vi "VI CG-Check Konfig.vi"() -> ()   [LabVIEW 2020, in "Erweiterte Konfig.lvlib" / "CG-Check Konfig.lvlib"]
uses:
  CG-Check Konfig.lvlib
  Sollwerte_CG-Check.ctl
  Komponenten.ctl
  maxAbweichung_CG-Check.ctl
  Visualisierungs Elemente/Auswahlfeld.ctl
  System Einstellungen V2/Gasflasche Auswahl.ctl
  System Einstellungen V2/Konfig Gasflasche.ctl
  Analysator Definition/FGV Analysator Definition Aktionen.ctl
  System Einstellungen V2/Aktioen FGV System Konstanten.ctl
  System Einstellungen V2/Aktion FGV Gasbottledefinition.ctl
  FT-IR/FGV FT-IR Gasliste Aktionen.ctl
  CalEingaenge.ctl
  Aktion_CG-Check.ctl
  CG-Test.vi
  FT-IR/FT-IR.lvlib
  Allgemein/allgemeine Sub-VIs.lvlib
  Analysator Definition/Analysator Definition.lvlib
  Sprachverwaltung/Sprachverwaltung.lvlib
  System Einstellungen V2/System Einstellungen V2.lvlib
panel:
  in  "Start":bool
  in  "Auswertung":bool caption="Ergebnis"
  in  "Textname:":string
  in  "Pfad:":path=path "D:/IAG_Data/Log" caption="Pfad CalGas Test:"
  in  "Cluster":T1={"Aufschaltdauer"=0.0, "Prüfdauer"=0.0, "Mittelwertanzahl"=10} {"Prüfdauer" format="%#_5g"; "Aufschaltdauer" format="%#_5g"}
  in  "CalGas Konfig":T2(tab)
  in  "Konfig Gasflasche 1":T3 caption="Konfigurierte Gasflasche verwenden"
  in  "Gasflasche 1":T4 caption="Gasflasche" items=["----"=10000]
  in  "Analysator 1":T5 caption="Analysator"
  in  "über PNS":bool
  in  "Komponenten 1":T6 caption="Komponente" {"Komponente 5" items=["---"]; "Komponente 4" items=["---"]; "Komponente 3" items=["---"]; "Komponente 2" items=["---"]; "Komponente 1" items=["---"]}
  in  "Sollwerte 1":T7 caption="Sollwert" {"Sollwert 5" format="%#_10f"; "Sollwert 4" format="%#_10f"; "Sollwert 3" format="%#_10f"; "Sollwert 2" format="%#_10f"; "Sollwert 1" format="%#_10f"}
  in  "max. Abweichung 1":T8 caption="max. Abweichung" {"Abweichung 5" format="%#_5g"; "Abweichung 4" format="%#_5g"; "Abweichung 3" format="%#_5g"; "Abweichung 2" format="%#_5g"; "Abweichung 1" format="%#_5g"}
  in  "Span 1 durchführen":bool
  in  "Konfig Gasflasche 2":T3 caption="Konfigurierte Gasflasche verwenden"
  in  "Gasflasche 2":T4 caption="Gasflasche" items=["----"=10000]
  in  "über PNS":bool
  in  "Sollwerte 2":T7 caption="Sollwert" {"Sollwert 5" format="%#_10f"; "Sollwert 4" format="%#_10f"; "Sollwert 3" format="%#_10f"; "Sollwert 2" format="%#_10f"; "Sollwert 1" format="%#_10f"}
  in  "Komponenten 2":T6 caption="Komponente" {"Komponente 5" items=["---"]; "Komponente 4" items=["---"]; "Komponente 3" items=["---"]; "Komponente 2" items=["---"]; "Komponente 1" items=["---"]}
  in  "max. Abweichung 2":T8 caption="max. Abweichung" {"Abweichung 5" format="%#_5g"; "Abweichung 4" format="%#_5g"; "Abweichung 3" format="%#_5g"; "Abweichung 2" format="%#_5g"; "Abweichung 1" format="%#_5g"}
  in  "Span 2 durchführen":bool
  in  "Analysator 2":T5 caption="Analysator"
  in  "Konfig Gasflasche 3":T3 caption="Konfigurierte Gasflasche verwenden"
  in  "Gasflasche 3":T4 caption="Gasflasche" items=["----"=10000]
  in  "Sollwerte 3":T7 caption="Sollwert" {"Sollwert 5" format="%#_10f"; "Sollwert 4" format="%#_10f"; "Sollwert 3" format="%#_10f"; "Sollwert 2" format="%#_10f"; "Sollwert 1" format="%#_10f"}
  in  "Komponenten 3":T6 caption="Komponente" {"Komponente 5" items=["---"]; "Komponente 4" items=["---"]; "Komponente 3" items=["---"]; "Komponente 2" items=["---"]; "Komponente 1" items=["---"]}
  in  "max. Abweichung 3":T8 caption="max. Abweichung" {"Abweichung 5" format="%#_5g"; "Abweichung 4" format="%#_5g"; "Abweichung 3" format="%#_5g"; "Abweichung 2" format="%#_5g"; "Abweichung 1" format="%#_5g"}
  in  "über PNS":bool
  in  "Span 3 durchführen":bool
  in  "Analysator 3":T5 caption="Analysator"
  in  "Sollwerte 4":T7 caption="Sollwert" {"Sollwert 5" format="%#_10f"; "Sollwert 4" format="%#_10f"; "Sollwert 3" format="%#_10f"; "Sollwert 2" format="%#_10f"; "Sollwert 1" format="%#_10f"}
  in  "Komponenten 4":T6 caption="Komponente" {"Komponente 5" items=["---"]; "Komponente 4" items=["---"]; "Komponente 3" items=["---"]; "Komponente 2" items=["---"]; "Komponente 1" items=["---"]}
  in  "max. Abweichung 4":T8 caption="max. Abweichung" {"Abweichung 5" format="%#_5g"; "Abweichung 4" format="%#_5g"; "Abweichung 3" format="%#_5g"; "Abweichung 2" format="%#_5g"; "Abweichung 1" format="%#_5g"}
  in  "Cal Gas O2 durchführen":bool
  in  "Abbrechen":bool
  in  "speichern":bool
  in  "über PNS":bool caption="Span 1"
  # "Konfiguration CG-Test"
  # "sec"
  # "sec"
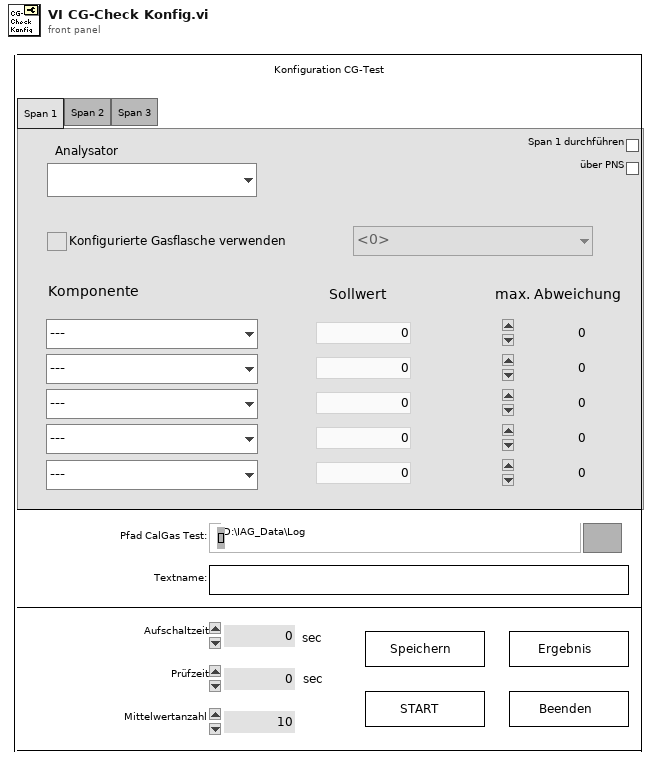
[diagram p1: front panel]
types:
  T1 = cluster{"Aufschaltdauer":sgl, "Prüfdauer":sgl, "Mittelwertanzahl":u8}
  T2 = enum32{"Span 1", "Span 2", "Span 3", "Cal Gas O2"}
  T3 = typedef "System Einstellungen V2.lvlib/Konfig Gasflasche.ctl" = bool
  T4 = typedef "System Einstellungen V2.lvlib/Gasflasche Auswahl.ctl" = u16
  T5 = typedef "Auswahlfeld.ctl" = u16
  T6 = typedef "Erweiterte Konfig.lvlib/CG-Check Konfig.lvlib/Komponenten.ctl" = cluster{"Komponente 1":u16, "Komponente 2":u16, "Komponente 3":u16, "Komponente 4":u16, "Komponente 5":u16}
  T7 = typedef "Erweiterte Konfig.lvlib/CG-Check Konfig.lvlib/Sollwerte_CG-Check.ctl" = cluster{"Sollwert 1":sgl, "Sollwert 2":sgl, "Sollwert 3":sgl, "Sollwert 4":sgl, "Sollwert 5":sgl}
  T8 = typedef "Erweiterte Konfig.lvlib/CG-Check Konfig.lvlib/maxAbweichung_CG-Check.ctl" = cluster{"Abweichung 1":sgl, "Abweichung 2":sgl, "Abweichung 3":sgl, "Abweichung 4":sgl, "Abweichung 5":sgl}
  T9 = typedef "System Einstellungen V2.lvlib/Aktion FGV Gasbottledefinition.ctl" = enum16{"lesen", "schreiben", "löschen", "laden", "speichern", "exportieren", "importieren"}
  T10 = typedef "System Einstellungen V2.lvlib/Aktioen FGV System Konstanten.ctl" = enum16{"lesen", "laden", "speichern", "Sprache"}
  T11 = typedef "Analysator Definition.lvlib/FGV Analysator Definition Aktionen.ctl" = enum16{"lesen", "MB setzen", "MB KAL setzen", "laden"}
  T12 = typedef "Erweiterte Konfig.lvlib/CG-Check Konfig.lvlib/Aktion_CG-Check.ctl" = enum16{"lesen", "schreiben", "laden", "Komponente", "Aktive?", "speichern"}
  T13 = typedef "Erweiterte Konfig.lvlib/CG-Check Konfig.lvlib/CalEingaenge.ctl" = string[]
  T14 = typedef "FT-IR.lvlib/FGV FT-IR Gasliste Aktionen.ctl" = enum16{"lesen", "Gasliste FT-IR", "Gasliste ausgelesen", "laden", "speichern", "löschen"}
  T15 = enum8{"Enabled", "Disabled", "Disabled and Grayed Out"}
  T16 = typedef "System Einstellungen V2.lvlib/Gasflasche gesamt.ctl" = cluster{"Gasflasche":T17, "Trägergas":T18, "Komponenten":T19[]}
  T17 = typedef "System Einstellungen V2.lvlib/Gasflasche.ctl" = cluster{"Gasname für die Auswahl":string, "Chargennummer":string, "Ablaufdatum":timestamp}
  T18 = typedef "System Einstellungen V2.lvlib/Traegergas.ctl" = string
  T19 = typedef "System Einstellungen V2.lvlib/Gasflaschenkomponente.ctl" = cluster{"Gasauswahl":string, "Konzentration IST":dbl, "Einheit":string, "Genauigkeit":dbl}
  T20 = typedef "String - Ausgabefeld.ctl" = string
  T21 = cluster{"Gasflasche":T4[], "Konfig Gasflasche":T3[]}
  T22 = cluster{"Komponenten[0]":u16, "Komponenten[1]":u16, "Komponenten[2]":u16, "Komponenten[3]":u16, "Komponenten[4]":u16}
  T23 = cluster{"max Abweichung[0]":sgl, "max Abweichung[1]":sgl, "max Abweichung[2]":sgl, "max Abweichung[3]":sgl, "max Abweichung[4]":sgl}
  T24 = cluster{"Sollwerte[0]":sgl, "Sollwerte[1]":sgl, "Sollwerte[2]":sgl, "Sollwerte[3]":sgl, "Sollwerte[4]":sgl}
  T25 = cluster{"[0]":i32, "[1]":i32, "[2]":i32, "[3]":i32, "[4]":i32}
  T26 = cluster{"[0]":dbl, "[1]":dbl, "[2]":dbl, "[3]":dbl, "[4]":dbl}
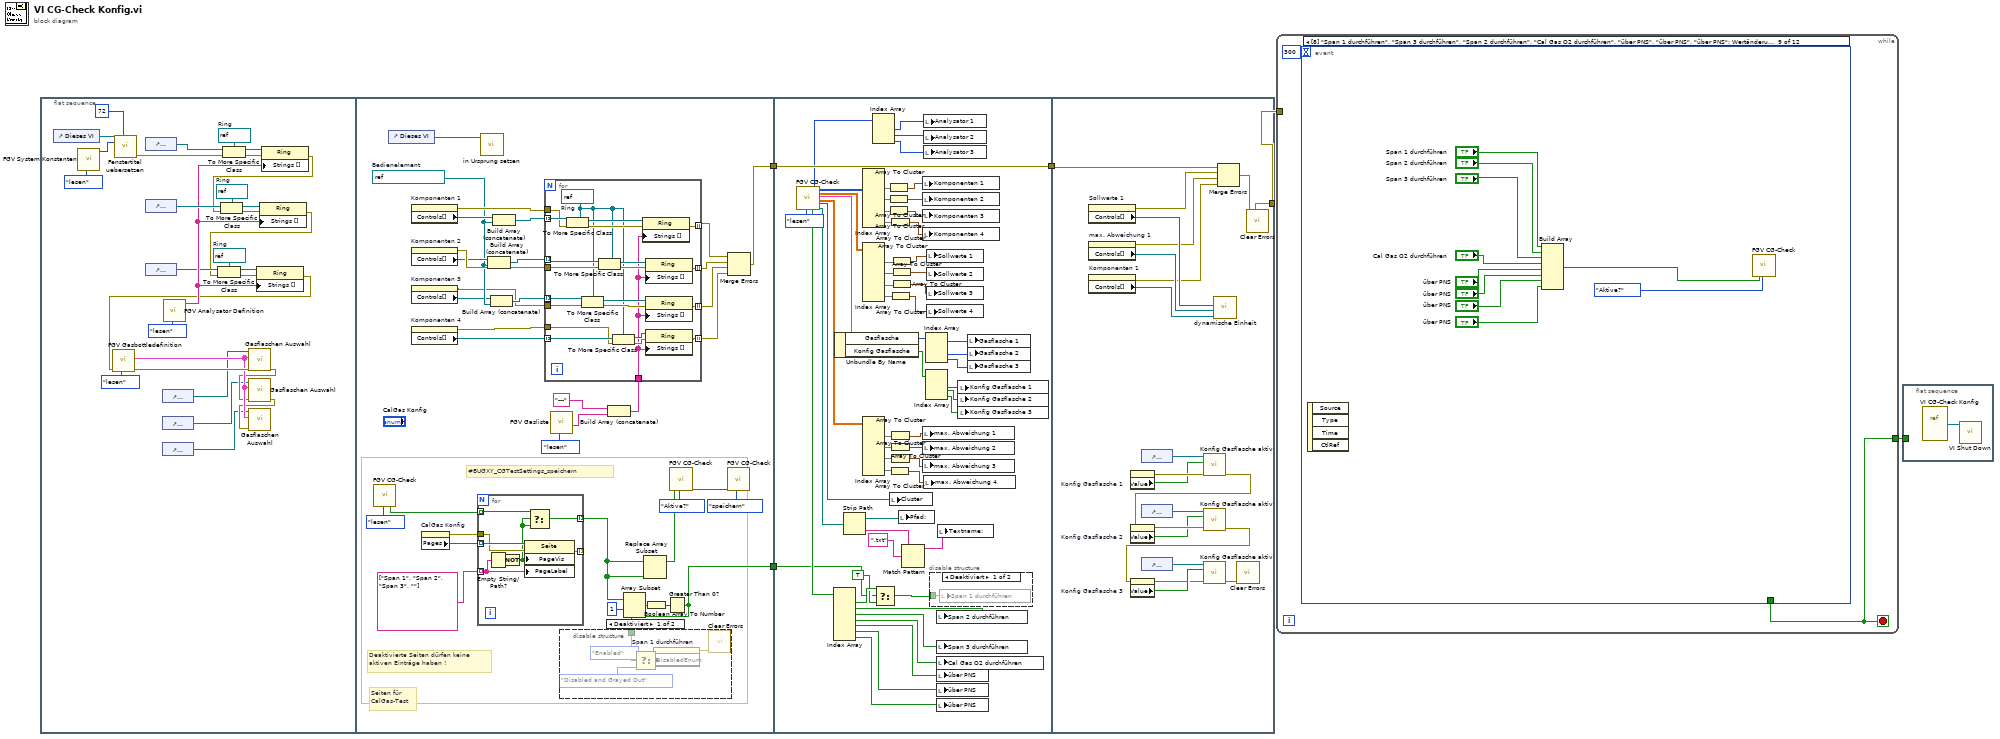
[diagram p0: block diagram]
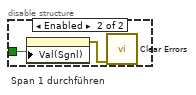
[diagram p3: hidden frame]
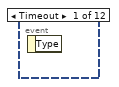
[diagram p4: hidden frame]
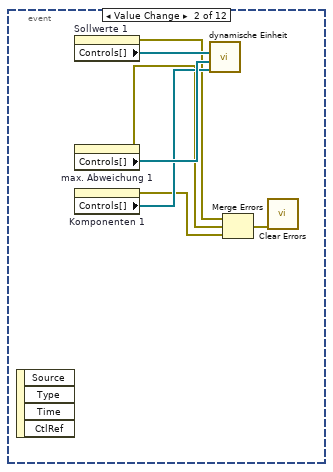
[diagram p5: hidden frame]
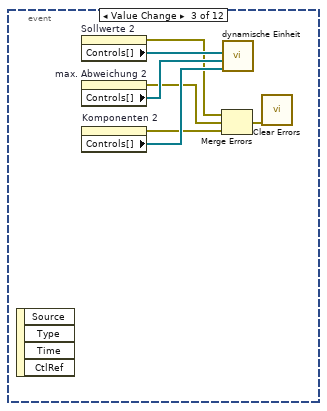
[diagram p6: hidden frame]
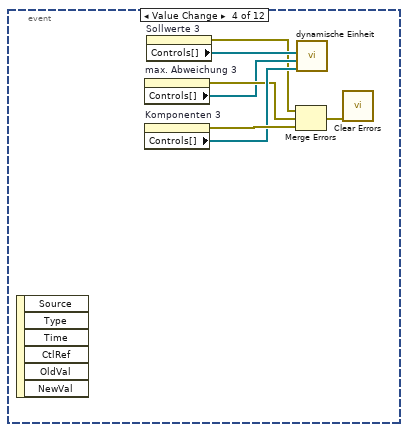
[diagram p7: hidden frame]
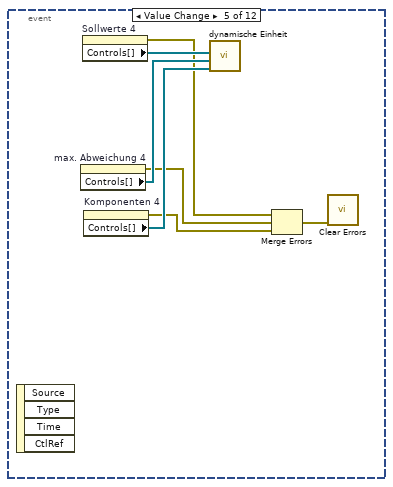
[diagram p8: hidden frame]
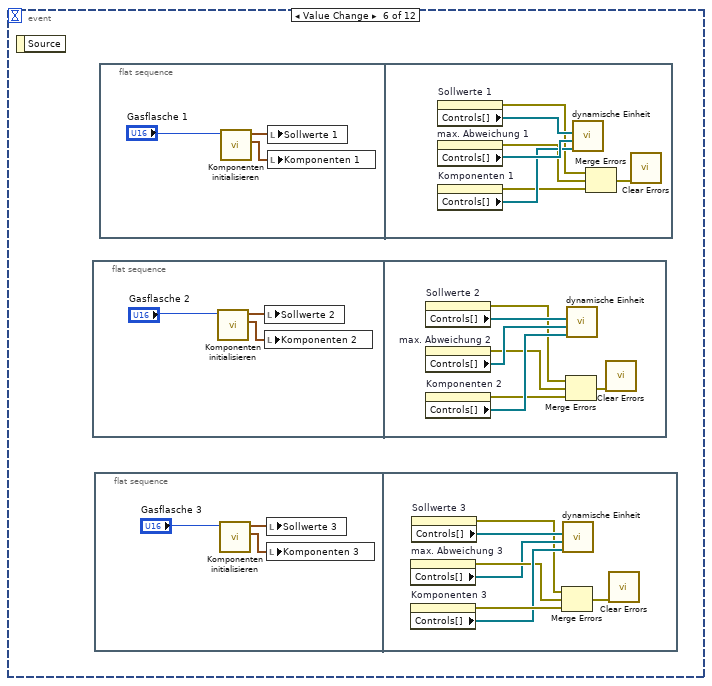
[diagram p9: hidden frame]
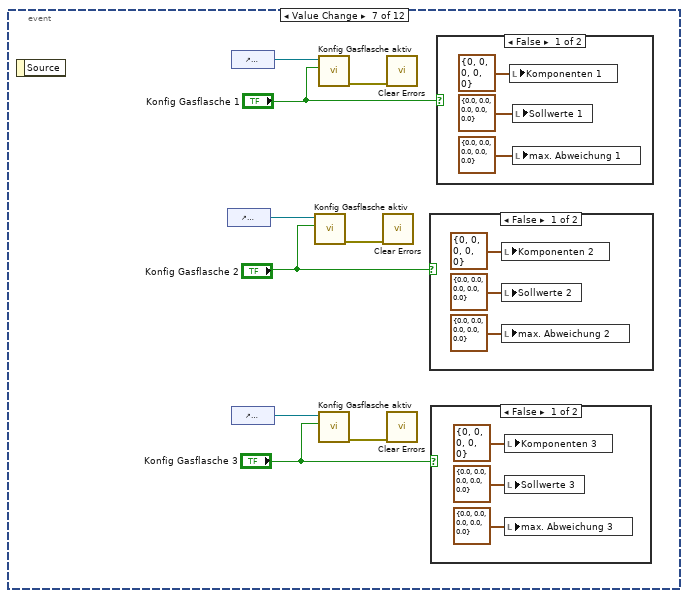
[diagram p10: hidden frame]
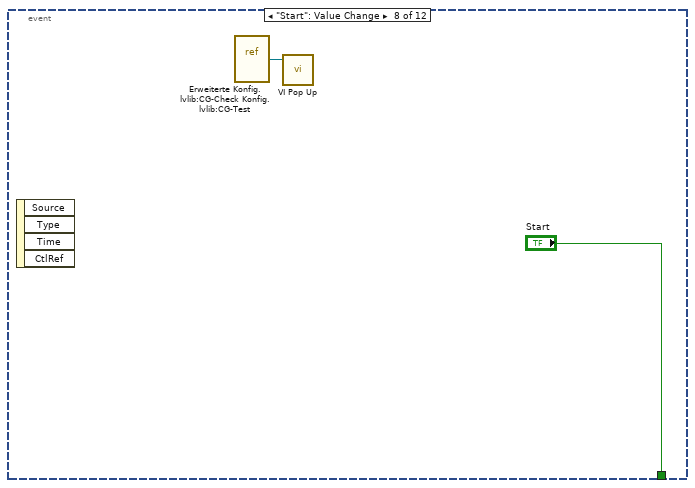
[diagram p14: hidden frame]
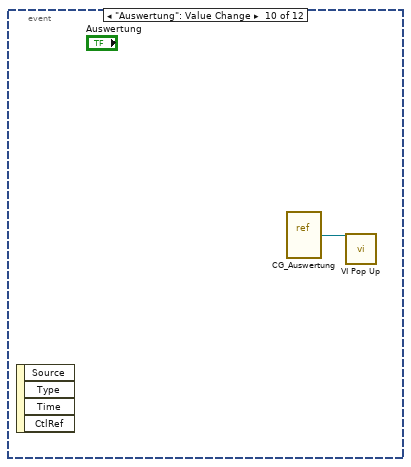
[diagram p15: hidden frame]
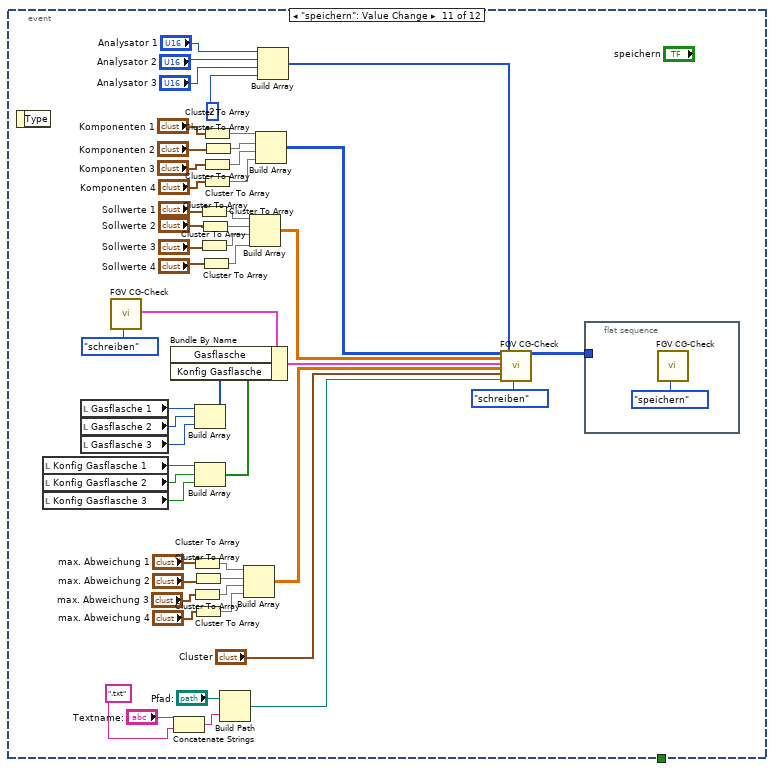
[diagram p16: hidden frame]
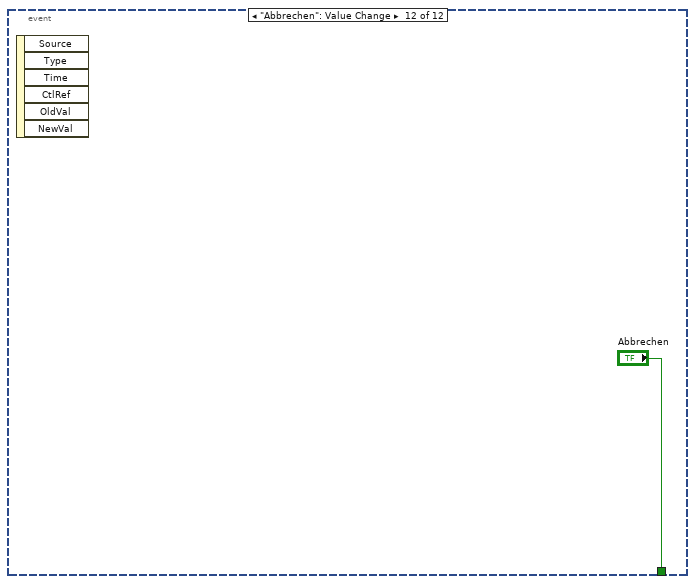
[diagram p17: hidden frame]
diagram:
  n1 = flat-sequence {
    tunnel: [w59] -> w3
    tunnel: [w42] -> w1
    tunnel: [w165] -> w4
    tunnel: w3 -> [w165]
    tunnel: w1 -> [w117]
    tunnel: w4 -> [w189]
    tunnel: [w188] -> w2
    frame #0 {
      w27 = refnum<vi> refnum  # Ring
      w30 = refnum<vi> refnum  # Ring
      w33 = refnum<vi> refnum  # Ring
      n2 = control-ref of="Dieses VI"() -> (w22:refnum<vi>)
      n3 = call "FGV System Konstanten.vi"("Aktionen"=Aktioen_FGV_System_Konstanten."lesen") -> ("Sprachindex"=w19:u16)  [unwired: 6 in, 4 out]
      n4 = call "Fenstertitel uebersetzen.vi"("Index (Seite)"=72, "Sprachauswahl"=w19, "Dieses VI"=w22) -> ("error out"=w9:errorcluster)  [unwired: 5 in, 3 out]
      n5 = control-ref of="Analysator 1"() -> (w18:refnum<vi>)
      n6 = control-ref of="Analysator 2"() -> (w25:refnum<vi>)
      n7 = control-ref of="Analysator 3"() -> (w23:refnum<vi>)
      n8 = control-ref of="Gasflasche 1"() -> (w12:refnum<vi>)
      n9 = control-ref of="Gasflasche 2"() -> (w11:refnum<vi>)
      n10 = control-ref of="Gasflasche 3"() -> (w10:refnum<vi>)
      n11 = call "FGV Analysator Definition.vi"("Aktionen"=FGV_Analysator_Definition_Aktionen."lesen") -> ("Analysatoren"=w24:string[])  [unwired: 6 in, 4 out]
      n12 = To More Specific Class(target class=w33, reference=w18, error in=w9) -> (specific class reference=w32:refnum<vi>, error out=w35:errorcluster)
      n13 = property class="Ring"(reference=w32, error in=w35, "Strings []"=w24) -> (error out=w8:errorcluster)  [unwired: 1 out]
      n14 = To More Specific Class(target class=w30, reference=w25, error in=w8) -> (specific class reference=w29:refnum<vi>, error out=w31:errorcluster)
      n15 = property class="Ring"(reference=w29, error in=w31, "Strings []"=w24) -> (error out=w7:errorcluster)  [unwired: 1 out]
      n16 = To More Specific Class(target class=w27, reference=w23, error in=w7) -> (specific class reference=w26:refnum<vi>, error out=w28:errorcluster)
      n17 = property class="Ring"(reference=w26, error in=w28, "Strings []"=w24) -> (error out=w6:errorcluster)  [unwired: 1 out]
      n18 = call "FGV Gasbottledefinition.vi"("Aktion"=Aktion_FGV_Gasbottledefinition."lesen", "error in (no error)"=w6) -> ("error out"=w16:errorcluster, "Gasflaschen Liste gesamt"=w15:T16[])  [unwired: 7 in, 1 out]
      n19 = call "Gasflaschen Auswahl.vi"("error in (no error)"=w16, "Gasflaschen Liste gesamt"=w15, "Ring (Eingang)"=w12) -> ("error out"=w14:errorcluster)  [unwired: 8 in]
      n20 = call "Gasflaschen Auswahl.vi"("error in (no error)"=w14, "Gasflaschen Liste gesamt"=w15, "Ring (Eingang)"=w11) -> ("error out"=w13:errorcluster)  [unwired: 8 in]
      n21 = call "Gasflaschen Auswahl.vi"("error in (no error)"=w13, "Gasflaschen Liste gesamt"=w15, "Ring (Eingang)"=w10) -> ()  [unwired: 8 in, 1 out]
    }
    frame #1 {
      w54 = refnum<vi> refnum  # Bedienelement
      # "#BUGXY_CGTestSettings_speichern"
      # "Deaktivierte Seiten dürfen keine \naktiven Einträge haben !"
      # "Seiten für \nCalGas-Test"
      n22 = call "FGV CG-Check.vi"("Aktion"=Aktion_CG-Check."lesen") -> ("Aktive?"=w37:bool[])  [unwired: 11 in, 7 out]
      n23 = control-ref of="Dieses VI"() -> (w71:refnum<vi>)
      n24 = property on="Komponenten 1" class="Cluster (strikt)"() -> (error out=w66:errorcluster, "Controls[]"=w65:refnum<vi>[])  [unwired: 2 in, 1 out]
      n25 = property on="Komponenten 2" class="Cluster (strikt)"() -> (error out=w64:errorcluster, "Controls[]"=w63:refnum<vi>[])  [unwired: 2 in, 1 out]
      n26 = property on="Komponenten 3" class="Cluster (strikt)"() -> (error out=w39:errorcluster, "Controls[]"=w38:refnum<vi>[])  [unwired: 2 in, 1 out]
      n27 = property on="Komponenten 4" class="Cluster (strikt)"() -> (error out=w40:errorcluster, "Controls[]"=w41:refnum<vi>[])  [unwired: 2 in, 1 out]
      n28 = property on="CalGas Konfig" class="RKElem (strikt)"() -> (error out=w52:errorcluster, "Pages"=w53:refnum<vi>[])  [unwired: 2 in, 1 out]
      n29 = for {
        tunnel: w53 -> [w106] mode=indexing
        tunnel: w52 -> [w105]
        tunnel: [w104] -> _ mode=indexing
        tunnel: T13 ["Span 1", "Span 2", "Span 3", ""] -> [w103] mode=indexing
        tunnel: w37 -> [w101] mode=indexing
        tunnel: [w99] -> w36 mode=indexing
        n30 = Empty String/Path?(string/path=w103) -> (empty?=w102:bool)
        n31 = Not(x=w102) -> (.not. x?=w100:bool)
        n32 = property class="Seite"(reference=w106, error in=w105, "PageVis"=w100, "PageLabel"=w103) -> (error out=w104:errorcluster)  [unwired: 1 out]
        n33 = Select(t=w101, s=w100, f=w100) -> (s? t:f=w99:bool)
      }
      n34 = call "in Ursprung setzen.vi"("VI Referenz"=w71) -> ()  [unwired: 10 in, 1 out]
      n35 = Build Array (concatenate)(w63, w54) -> (w56:refnum<vi>[])
      n36 = Build Array (concatenate)(w38, w54) -> (w55:refnum<vi>[])
      n37 = Build Array (concatenate)(w65, w54) -> (w57:refnum<vi>[])
      n38 = call "FGV Gasliste.vi"("Aktionen"=FGV_FT-IR_Gasliste_Aktionen."lesen") -> ("Aktuelle Gasliste gesamt"=w67:T20[])  [unwired: 8 in, 2 out]
      n39 = Build Array (concatenate)("---" ("String"), w67) -> (w70:T20[])
      n40 = for {
        tunnel: w57 -> [w96] mode=indexing
        tunnel: [w95] -> w61 mode=indexing
        tunnel: w66 -> [w94]
        tunnel: w70 -> [w77]
        tunnel: w64 -> [w90]
        tunnel: w56 -> [w89] mode=indexing
        tunnel: w39 -> [w88]
        tunnel: w55 -> [w87] mode=indexing
        tunnel: [w85] -> w62 mode=indexing
        tunnel: [w84] -> w60 mode=indexing
        tunnel: w41 -> [w80] mode=indexing
        tunnel: [w81] -> w58 mode=indexing
        tunnel: w40 -> [w79]
        w78 = refnum<vi> refnum  # Ring
        n41 = To More Specific Class(target class=w78, reference=w96, error in=w94) -> (specific class reference=w97:refnum<vi>, error out=w98:errorcluster)
        n42 = To More Specific Class(target class=w78, reference=w87, error in=w88) -> (specific class reference=w91:refnum<vi>, error out=w92:errorcluster)
        n43 = To More Specific Class(target class=w78, reference=w89, error in=w90) -> (specific class reference=w93:refnum<vi>, error out=w86:errorcluster)
        n44 = To More Specific Class(target class=w78, reference=w80, error in=w79) -> (specific class reference=w83:refnum<vi>, error out=w82:errorcluster)
        n45 = property class="Ring"(reference=w97, error in=w98, "Strings []"=w77) -> (error out=w95:errorcluster)  [unwired: 1 out]
        n46 = property class="Ring"(reference=w93, error in=w86, "Strings []"=w77) -> (error out=w85:errorcluster)  [unwired: 1 out]
        n47 = property class="Ring"(reference=w91, error in=w92, "Strings []"=w77) -> (error out=w84:errorcluster)  [unwired: 1 out]
        n48 = property class="Ring"(reference=w83, error in=w82, "Strings []"=w77) -> (error out=w81:errorcluster)  [unwired: 1 out]
      }
      n49 = Array Subset(array=w36, index=1 ("Index")) -> (w44:bool[])  [unwired: 1 in]
      n50 = Replace Array Subset(array=w36, new element=w36) -> (w49:bool[])  [unwired: 1 in]
      n51 = Boolean Array To Number(Boolean array=w44) -> (number=w43:u32)
      n52 = Greater Than 0?(x=w43) -> (x > 0?=w42:bool)
      n53 = disable-structure shown="Deaktiviert" {
        disable-tunnel: w42 -> [w72 _]
        frame Disabled {
          n54 = Select(t=T15."Enabled" ("Deaktiviert"), s=w72, f=T15."Disabled and Grayed Out" ("Deaktiviert")) -> (s? t:f=w75:T15)
          n55 = property on="Span 1 durchführen" class="Bool. (strikt)"("DisabledEnum"=w75) -> (error out=w76:errorcluster)  [unwired: 2 in, 1 out]
          n56 = call <vilib>:"Clear Errors.vi"("error in (no error)"=w76) -> ()  [unwired: 5 in, 2 out]
        }
        frame Enabled {
        }
      }
      n57 = call "FGV CG-Check.vi"("Aktive?"=w49, "Aktion"=Aktion_CG-Check."Aktive?") -> ("Pfad:"=w48:path)  [unwired: 10 in, 7 out]
      n58 = call "FGV CG-Check.vi"("Pfad:"=w48, "Aktion"=Aktion_CG-Check."speichern") -> ()  [unwired: 10 in, 8 out]
      n59 = Merge Errors(w61, w62, w60, w58) -> (w59:errorcluster)
    }
    frame #2 {
      n60 = call "FGV CG-Check.vi"("Aktion"=Aktion_CG-Check."lesen") -> ("Analysator"=w123:T5[], "Aktive?"=w133:bool[], "Komponenten"=w162:u16[][], "Sollwerte"=w155:sgl[][], "Gaskonfig"=w115:T21, "max Abweichung"=w154:sgl[][], "Cluster"=w163:T1, "Pfad:"=w143:path)  [unwired: 11 in]
      n61 = Index Array(array=w133) -> (element #1=w119:bool, element #2=w132:bool, element #3=w131:bool, element #4=w130:bool, element #5=w126:bool, element #6=w125:bool, element #7=w124:bool)  [unwired: 7 in]
      n62 = Unbundle By Name(w115) -> ("Gasflasche"=w114:T4[], "Konfig Gasflasche"=w113:T3[])
      n63 = Strip Path(path=w143) -> (stripped path=w142:path, name=w141:string)
      n64 = Index Array(array=w162) -> (element #1=w161:u16[], element #2=w160:u16[], element #3=w159:u16[], element #4=w136:u16[])  [unwired: 8 in]
      n65 = Index Array(array=w155) -> (element #1=w153:sgl[], element #2=w152:sgl[], element #3=w151:sgl[], element #4=w135:sgl[])  [unwired: 8 in]
      n66 = Index Array(array=w154) -> (element #1=w150:sgl[], element #2=w149:sgl[], element #3=w148:sgl[], element #4=w134:sgl[])  [unwired: 8 in]
      n67 = Index Array(array=w123) -> (element #1=w122:T5, element #2=w121:T5, element #3=w120:T5)  [unwired: 3 in]
      n68 = Select(t=w119, s=w117, f=TRUE ("t")) -> (s? t:f=w116:bool)
      n69 = Array To Cluster(array=w161) -> (cluster=w157:T22)
      n70 = Array To Cluster(array=w160) -> (cluster=w158:T22)
      n71 = Array To Cluster(array=w159) -> (cluster=w156:T22)
      n72 = Array To Cluster(array=w134) -> (cluster=w129:T23)
      n73 = Array To Cluster(array=w136) -> (cluster=w127:T22)
      n74 = Array To Cluster(array=w150) -> (cluster=w146:T23)
      n75 = Array To Cluster(array=w149) -> (cluster=w144:T23)
      n76 = Array To Cluster(array=w148) -> (cluster=w145:T23)
      n77 = Array To Cluster(array=w135) -> (cluster=w128:T24)
      n78 = local write "Cluster"(w163) -> ()
      n79 = Array To Cluster(array=w153) -> (cluster=w147:T24)
      n80 = Array To Cluster(array=w152) -> (cluster=w138:T24)
      n81 = Array To Cluster(array=w151) -> (cluster=w137:T24)
      n82 = local write "Pfad:"(w142) -> ()
      n83 = Match Pattern(string=w141, regular expression=".txt" ("Regulärer Ausdruck")) -> (before substring=w139:string)  [unwired: 1 in, 3 out]
      n84 = local write "Komponenten 1"(w157) -> ()
      n85 = local write "Komponenten 2"(w158) -> ()
      n86 = local write "Komponenten 3"(w156) -> ()
      n87 = local write "Komponenten 4"(w127) -> ()
      n88 = local write "max. Abweichung 1"(w146) -> ()
      n89 = local write "max. Abweichung 2"(w144) -> ()
      n90 = local write "max. Abweichung 3"(w145) -> ()
      n91 = local write "Analysator 1"(w122) -> ()
      n92 = local write "Analysator 2"(w121) -> ()
      n93 = local write "Analysator 3"(w120) -> ()
      n94 = local write "max. Abweichung 4"(w129) -> ()
      n95 = Index Array(array=w114) -> (element #1=w112:T4, element #2=w111:T4, element #3=w110:T4)  [unwired: 3 in]
      n96 = Index Array(array=w113) -> (element #1=w109:T3, element #2=w108:T3, element #3=w107:T3)  [unwired: 3 in]
      n97 = local write "Sollwerte 1"(w147) -> ()
      n98 = local write "Sollwerte 2"(w138) -> ()
      n99 = local write "Sollwerte 3"(w137) -> ()
      n100 = local write "Sollwerte 4"(w128) -> ()
      n101 = disable-structure shown="Deaktiviert" {
        disable-tunnel: w116 -> [w166 w167]
        frame Disabled {
          n102 = local write "Span 1 durchführen"(w166) -> ()
        }
        frame Enabled {
          n103 = property on="Span 1 durchführen" class="Bool. (strikt)"("Val(Sgnl)"=w167) -> (error out=w168:errorcluster)  [unwired: 2 in, 1 out]
          n104 = call <vilib>:"Clear Errors.vi"("error in (no error)"=w168) -> ()  [unwired: 5 in, 2 out]
        }
      }
      n105 = local write "Span 2 durchführen"(w132) -> ()
      n106 = local write "Span 3 durchführen"(w131) -> ()
      n107 = local write "Cal Gas O2 durchführen"(w130) -> ()
      n108 = local write "über PNS"(w126) -> ()
      n109 = local write "über PNS"(w125) -> ()
      n110 = local write "über PNS"(w124) -> ()
      n111 = local write "Textname:"(w139) -> ()
      n112 = local write "Konfig Gasflasche 1"(w109) -> ()
      n113 = local write "Konfig Gasflasche 2"(w108) -> ()
      n114 = local write "Konfig Gasflasche 3"(w107) -> ()
      n115 = local write "Gasflasche 1"(w112) -> ()
      n116 = local write "Gasflasche 2"(w111) -> ()
      n117 = local write "Gasflasche 3"(w110) -> ()
    }
    frame #3 {
      n118 = property on="Sollwerte 1" class="Cluster (strikt)"() -> (error out=w181:errorcluster, "Controls[]"=w185:refnum<vi>[])  [unwired: 2 in, 1 out]
      n119 = property on="max. Abweichung 1" class="Cluster (strikt)"() -> (error out=w183:errorcluster, "Controls[]"=w184:refnum<vi>[])  [unwired: 2 in, 1 out]
      n120 = property on="Komponenten 1" class="Cluster (strikt)"() -> (error out=w182:errorcluster, "Controls[]"=w186:refnum<vi>[])  [unwired: 2 in, 1 out]
      n121 = property on="Konfig Gasflasche 1" class="Bool. (strikt)"() -> (error out=w171:errorcluster, "Value"=w170:T3)  [unwired: 2 in, 1 out]
      n122 = control-ref of="Gasflasche 1"() -> (w178:refnum<vi>)
      n123 = control-ref of="Gasflasche 2"() -> (w179:refnum<vi>)
      n124 = control-ref of="Gasflasche 3"() -> (w180:refnum<vi>)
      n125 = call "Konfig Gasflasche aktiv.vi"("error in (no error)"=w171, "Konfig Gasflasche"=w170, "Referenz Gasflasche"=w178) -> ("error out"=w176:errorcluster)  [unwired: 8 in]
      n126 = property on="Konfig Gasflasche 2" class="Bool. (strikt)"(error in=w176) -> (error out=w173:errorcluster, "Value"=w172:T3)  [unwired: 1 in, 1 out]
      n127 = call "Konfig Gasflasche aktiv.vi"("error in (no error)"=w173, "Konfig Gasflasche"=w172, "Referenz Gasflasche"=w179) -> ("error out"=w177:errorcluster)  [unwired: 8 in]
      n128 = property on="Konfig Gasflasche 3" class="Bool. (strikt)"(error in=w177) -> (error out=w174:errorcluster, "Value"=w175:T3)  [unwired: 1 in, 1 out]
      n129 = call "Konfig Gasflasche aktiv.vi"("error in (no error)"=w174, "Konfig Gasflasche"=w175, "Referenz Gasflasche"=w180) -> ("error out"=w169:errorcluster)  [unwired: 8 in]
      n130 = call "dynamische Einheit.vi"("Komponenten Ref."=w186, "max.Abweichung Ref."=w184, "Sollwert Ref."=w185) -> ()  [unwired: 9 in]
      n131 = Merge Errors(w189, w181, w183, w182) -> (w187:errorcluster)
      n132 = call <vilib>:"Clear Errors.vi"("error in (no error)"=w169) -> ()  [unwired: 5 in, 2 out]
      n133 = call <vilib>:"Clear Errors.vi"("error in (no error)"=w187) -> ("error out"=w188:errorcluster)  [unwired: 5 in, 1 out]
    }
  }
  n134 = while {
    tunnel: [w190] -> w5
    tunnel: w2 -> [_]
    stop <- w190 stop-if-true
    n135 = event shown="[8] \"Span 1 durchführen\", \"Span 3 durchführen\", \"Span 2 durchführen\", \"Cal Gas O2 durchführen\", \"über PNS\", \"über PNS\", \"über PNS\": Wertänderung" {
      selector: _ -> [_ _ _ _ _ _ _ _ _ _ _ _]
      dyn-events: _ -> [_ _ _ _ _ _ _ _ _ _ _ _]
      timeout: 300 -> [_ _ _ _ _ _ _ _ _ _ _ _]
      tunnel: [_ _ _ _ _ _ _ "Start" _ _ _ "Abbrechen"] -> w190
      event Timeout {
        n136 = event-data() -> ()  [unwired: 1 in, 1 out]
      }
      event Value Change {
        n137 = event-data() -> ()  [unwired: 1 in, 4 out]
        n138 = property on="Sollwerte 1" class="Cluster (strikt)"() -> (error out=w194:errorcluster, "Controls[]"=w198:refnum<vi>[])  [unwired: 2 in, 1 out]
        n139 = property on="max. Abweichung 1" class="Cluster (strikt)"() -> (error out=w193:errorcluster, "Controls[]"=w197:refnum<vi>[])  [unwired: 2 in, 1 out]
        n140 = property on="Komponenten 1" class="Cluster (strikt)"() -> (error out=w192:errorcluster, "Controls[]"=w196:refnum<vi>[])  [unwired: 2 in, 1 out]
        n141 = call "dynamische Einheit.vi"("Komponenten Ref."=w196, "max.Abweichung Ref."=w197, "Sollwert Ref."=w198) -> ()  [unwired: 9 in]
        n142 = Merge Errors(w194, w193, w192) -> (w195:errorcluster)
        n143 = call <vilib>:"Clear Errors.vi"("error in (no error)"=w195) -> ()  [unwired: 5 in, 2 out]
      }
      event Value Change {
        n144 = event-data() -> ()  [unwired: 1 in, 4 out]
        n145 = property on="Sollwerte 2" class="Cluster (strikt)"() -> (error out=w201:errorcluster, "Controls[]"=w205:refnum<vi>[])  [unwired: 2 in, 1 out]
        n146 = property on="max. Abweichung 2" class="Cluster (strikt)"() -> (error out=w200:errorcluster, "Controls[]"=w204:refnum<vi>[])  [unwired: 2 in, 1 out]
        n147 = property on="Komponenten 2" class="Cluster (strikt)"() -> (error out=w199:errorcluster, "Controls[]"=w203:refnum<vi>[])  [unwired: 2 in, 1 out]
        n148 = Merge Errors(w201, w200, w199) -> (w202:errorcluster)
        n149 = call "dynamische Einheit.vi"("Komponenten Ref."=w203, "max.Abweichung Ref."=w204, "Sollwert Ref."=w205) -> ()  [unwired: 9 in]
        n150 = call <vilib>:"Clear Errors.vi"("error in (no error)"=w202) -> ()  [unwired: 5 in, 2 out]
      }
      event Value Change {
        n151 = event-data() -> ()  [unwired: 1 in, 6 out]
        n152 = property on="max. Abweichung 3" class="Cluster (strikt)"() -> (error out=w209:errorcluster, "Controls[]"=w208:refnum<vi>[])  [unwired: 2 in, 1 out]
        n153 = property on="Komponenten 3" class="Cluster (strikt)"() -> (error out=w211:errorcluster, "Controls[]"=w210:refnum<vi>[])  [unwired: 2 in, 1 out]
        n154 = property on="Sollwerte 3" class="Cluster (strikt)"() -> (error out=w206:errorcluster, "Controls[]"=w207:refnum<vi>[])  [unwired: 2 in, 1 out]
        n155 = Merge Errors(w206, w209, w211) -> (w212:errorcluster)
        n156 = call "dynamische Einheit.vi"("Komponenten Ref."=w210, "max.Abweichung Ref."=w208, "Sollwert Ref."=w207) -> ()  [unwired: 9 in]
        n157 = call <vilib>:"Clear Errors.vi"("error in (no error)"=w212) -> ()  [unwired: 5 in, 2 out]
      }
      event Value Change {
        n158 = event-data() -> ()  [unwired: 1 in, 4 out]
        n159 = property on="max. Abweichung 4" class="Cluster (strikt)"() -> (error out=w214:errorcluster, "Controls[]"=w217:refnum<vi>[])  [unwired: 2 in, 1 out]
        n160 = property on="Sollwerte 4" class="Cluster (strikt)"() -> (error out=w215:errorcluster, "Controls[]"=w218:refnum<vi>[])  [unwired: 2 in, 1 out]
        n161 = property on="Komponenten 4" class="Cluster (strikt)"() -> (error out=w213:errorcluster, "Controls[]"=w216:refnum<vi>[])  [unwired: 2 in, 1 out]
        n162 = call "dynamische Einheit.vi"("Komponenten Ref."=w216, "max.Abweichung Ref."=w217, "Sollwert Ref."=w218) -> ()  [unwired: 9 in]
        n163 = Merge Errors(w215, w214, w213) -> (w219:errorcluster)
        n164 = call <vilib>:"Clear Errors.vi"("error in (no error)"=w219) -> ()  [unwired: 5 in, 2 out]
      }
      event Value Change {
        n165 = event-data() -> ()  [unwired: 1 in, 1 out]
        n166 = flat-sequence {
          frame #0 {
            n167 = call "Komponenten initialisieren.vi"("Gasflasche"="Gasflasche 2") -> ("Komponente"=w231:T25, "Sollwerte"=w232:T26)  [unwired: 9 in]
            n168 = local write "Sollwerte 2"(w232) -> ()
            n169 = local write "Komponenten 2"(w231) -> ()
          }
          frame #1 {
            n170 = property on="Sollwerte 2" class="Cluster (strikt)"() -> (error out=w235:errorcluster, "Controls[]"=w239:refnum<vi>[])  [unwired: 2 in, 1 out]
            n171 = property on="max. Abweichung 2" class="Cluster (strikt)"() -> (error out=w234:errorcluster, "Controls[]"=w238:refnum<vi>[])  [unwired: 2 in, 1 out]
            n172 = property on="Komponenten 2" class="Cluster (strikt)"() -> (error out=w233:errorcluster, "Controls[]"=w237:refnum<vi>[])  [unwired: 2 in, 1 out]
            n173 = Merge Errors(w235, w234, w233) -> (w236:errorcluster)
            n174 = call "dynamische Einheit.vi"("Komponenten Ref."=w237, "max.Abweichung Ref."=w238, "Sollwert Ref."=w239) -> ()  [unwired: 9 in]
            n175 = call <vilib>:"Clear Errors.vi"("error in (no error)"=w236) -> ()  [unwired: 5 in, 2 out]
          }
        }
        n176 = flat-sequence {
          frame #0 {
            n177 = call "Komponenten initialisieren.vi"("Gasflasche"="Gasflasche 3") -> ("Komponente"=w221:T25, "Sollwerte"=w222:T26)  [unwired: 9 in]
            n178 = local write "Sollwerte 3"(w222) -> ()
            n179 = local write "Komponenten 3"(w221) -> ()
          }
          frame #1 {
            n180 = property on="max. Abweichung 3" class="Cluster (strikt)"() -> (error out=w226:errorcluster, "Controls[]"=w225:refnum<vi>[])  [unwired: 2 in, 1 out]
            n181 = property on="Komponenten 3" class="Cluster (strikt)"() -> (error out=w228:errorcluster, "Controls[]"=w227:refnum<vi>[])  [unwired: 2 in, 1 out]
            n182 = property on="Sollwerte 3" class="Cluster (strikt)"() -> (error out=w223:errorcluster, "Controls[]"=w224:refnum<vi>[])  [unwired: 2 in, 1 out]
            n183 = Merge Errors(w223, w226, w228) -> (w229:errorcluster)
            n184 = call "dynamische Einheit.vi"("Komponenten Ref."=w227, "max.Abweichung Ref."=w225, "Sollwert Ref."=w224) -> ()  [unwired: 9 in]
            n185 = call <vilib>:"Clear Errors.vi"("error in (no error)"=w229) -> ()  [unwired: 5 in, 2 out]
          }
        }
        n186 = flat-sequence {
          frame #0 {
            n187 = call "Komponenten initialisieren.vi"("Gasflasche"="Gasflasche 1") -> ("Komponente"=w240:T25, "Sollwerte"=w241:T26)  [unwired: 9 in]
            n188 = local write "Sollwerte 1"(w241) -> ()
            n189 = local write "Komponenten 1"(w240) -> ()
          }
          frame #1 {
            n190 = property on="Sollwerte 1" class="Cluster (strikt)"() -> (error out=w245:errorcluster, "Controls[]"=w249:refnum<vi>[])  [unwired: 2 in, 1 out]
            n191 = property on="max. Abweichung 1" class="Cluster (strikt)"() -> (error out=w244:errorcluster, "Controls[]"=w248:refnum<vi>[])  [unwired: 2 in, 1 out]
            n192 = property on="Komponenten 1" class="Cluster (strikt)"() -> (error out=w243:errorcluster, "Controls[]"=w247:refnum<vi>[])  [unwired: 2 in, 1 out]
            n193 = call "dynamische Einheit.vi"("Komponenten Ref."=w247, "max.Abweichung Ref."=w248, "Sollwert Ref."=w249) -> ()  [unwired: 9 in]
            n194 = Merge Errors(w245, w244, w243) -> (w246:errorcluster)
            n195 = call <vilib>:"Clear Errors.vi"("error in (no error)"=w246) -> ()  [unwired: 5 in, 2 out]
          }
        }
      }
      event Value Change {
        n196 = event-data() -> ()  [unwired: 1 in, 1 out]
        n197 = control-ref of="Gasflasche 2"() -> (w255:refnum<vi>)
        n198 = control-ref of="Gasflasche 1"() -> (w258:refnum<vi>)
        n199 = control-ref of="Gasflasche 3"() -> (w252:refnum<vi>)
        n200 = call "Konfig Gasflasche aktiv.vi"("Konfig Gasflasche"="Konfig Gasflasche 2", "Referenz Gasflasche"=w255) -> ("error out"=w254:errorcluster)  [unwired: 9 in]
        n201 = call "Konfig Gasflasche aktiv.vi"("Konfig Gasflasche"="Konfig Gasflasche 1", "Referenz Gasflasche"=w258) -> ("error out"=w257:errorcluster)  [unwired: 9 in]
        n202 = call "Konfig Gasflasche aktiv.vi"("Konfig Gasflasche"="Konfig Gasflasche 3", "Referenz Gasflasche"=w252) -> ("error out"=w251:errorcluster)  [unwired: 9 in]
        n203 = call <vilib>:"Clear Errors.vi"("error in (no error)"=w254) -> ()  [unwired: 5 in, 2 out]
        n204 = call <vilib>:"Clear Errors.vi"("error in (no error)"=w257) -> ()  [unwired: 5 in, 2 out]
        n205 = call <vilib>:"Clear Errors.vi"("error in (no error)"=w251) -> ()  [unwired: 5 in, 2 out]
        n206 = case shown="False" "Konfig Gasflasche 2" {
          frame False {
            n207 = local write "Komponenten 2"(T6 {"Komponente 1"=0, "Komponente 2"=0, "Komponente 3"=0, "Komponente 4"=0, "Komponente 5"=0} ("Komponenten 1")) -> ()
            n208 = local write "Sollwerte 2"(T7 {"Sollwert 1"=0.0, "Sollwert 2"=0.0, "Sollwert 3"=0.0, "Sollwert 4"=0.0, "Sollwert 5"=0.0} ("Sollwerte 1")) -> ()
            n209 = local write "max. Abweichung 2"(T8 {"Abweichung 1"=0.0, "Abweichung 2"=0.0, "Abweichung 3"=0.0, "Abweichung 4"=0.0, "Abweichung 5"=0.0} ("max. Abweichung 1")) -> ()
          }
          frame True {
          }
        }
        n210 = case shown="False" "Konfig Gasflasche 3" {
          frame False {
            n211 = local write "Komponenten 3"(T6 {"Komponente 1"=0, "Komponente 2"=0, "Komponente 3"=0, "Komponente 4"=0, "Komponente 5"=0} ("Komponenten 1")) -> ()
            n212 = local write "Sollwerte 3"(T7 {"Sollwert 1"=0.0, "Sollwert 2"=0.0, "Sollwert 3"=0.0, "Sollwert 4"=0.0, "Sollwert 5"=0.0} ("Sollwerte 1")) -> ()
            n213 = local write "max. Abweichung 3"(T8 {"Abweichung 1"=0.0, "Abweichung 2"=0.0, "Abweichung 3"=0.0, "Abweichung 4"=0.0, "Abweichung 5"=0.0} ("max. Abweichung 1")) -> ()
          }
          frame True {
          }
        }
        n214 = case shown="False" "Konfig Gasflasche 1" {
          frame False {
            n215 = local write "Komponenten 1"(T6 {"Komponente 1"=0, "Komponente 2"=0, "Komponente 3"=0, "Komponente 4"=0, "Komponente 5"=0} ("Komponenten 1")) -> ()
            n216 = local write "Sollwerte 1"(T7 {"Sollwert 1"=0.0, "Sollwert 2"=0.0, "Sollwert 3"=0.0, "Sollwert 4"=0.0, "Sollwert 5"=0.0} ("Sollwerte 1")) -> ()
            n217 = local write "max. Abweichung 1"(T8 {"Abweichung 1"=0.0, "Abweichung 2"=0.0, "Abweichung 3"=0.0, "Abweichung 4"=0.0, "Abweichung 5"=0.0} ("max. Abweichung 1")) -> ()
          }
          frame True {
          }
        }
      }
      event "Start": Value Change {
        n218 = event-data() -> ()  [unwired: 1 in, 4 out]
        n219 = vi-ref "Erweiterte Konfig.lvlib:CG-Check Konfig.lvlib:CG-Test.vi"() -> (w269:refnum<vi>)
        n220 = call "VI Pop Up.vi"("VI Referenz"=w269) -> ()  [unwired: 10 in, 1 out]
      }
      event "Span 1 durchführen", "Span 3 durchführen", "Span 2 durchführen", "Cal Gas O2 durchführen", "über PNS", "über PNS", "über PNS": Value Change {
        n221 = event-data() -> ()  [unwired: 1 in, 4 out]
        n222 = Build Array("Span 1 durchführen", "Span 2 durchführen", "Span 3 durchführen", "Cal Gas O2 durchführen", "über PNS", "über PNS", "über PNS", "über PNS") -> (w276:bool[])
        n223 = call "FGV CG-Check.vi"("Aktive?"=w276, "Aktion"=Aktion_CG-Check."Aktive?") -> ()  [unwired: 10 in, 8 out]
      }
      event "Auswertung": Value Change {
        n224 = event-data() -> ()  [unwired: 1 in, 4 out]
        n225 = vi-ref "CG_Auswertung.vi"() -> (w280:refnum<vi>)
        n226 = call "VI Pop Up.vi"("VI Referenz"=w280) -> ()  [unwired: 10 in, 1 out]
      }
      event "speichern": Value Change {
        n227 = event-data() -> ()  [unwired: 1 in, 1 out]
        n228 = local read "Konfig Gasflasche 1"() -> (w289:T3)
        n229 = local read "Konfig Gasflasche 2"() -> (w288:T3)
        n230 = local read "Konfig Gasflasche 3"() -> (w287:T3)
        n231 = local read "Gasflasche 1"() -> (w292:T4)
        n232 = local read "Gasflasche 2"() -> (w291:T4)
        n233 = local read "Gasflasche 3"() -> (w290:T4)
        n234 = call "FGV CG-Check.vi"("Aktion"=Aktion_CG-Check."schreiben") -> ("Gaskonfig"=w282:T21)  [unwired: 11 in, 7 out]
        n235 = Concatenate Strings("Textname:", ".txt") -> (w309:string)
        n236 = Cluster To Array(cluster="max. Abweichung 1") -> (array=w318:sgl[])
        n237 = Cluster To Array(cluster="max. Abweichung 3") -> (array=w319:sgl[])
        n238 = Cluster To Array(cluster="max. Abweichung 2") -> (array=w317:sgl[])
        n239 = Cluster To Array(cluster="max. Abweichung 4") -> (array=w301:sgl[])
        n240 = Build Array(w292, w291, w290) -> (w286:T4[])
        n241 = Build Array(w289, w288, w287) -> (w285:T3[])
        n242 = Bundle By Name(cluster=w282, "Gasflasche"=w286, "Konfig Gasflasche"=w285) -> (w284:T21)
        n243 = Cluster To Array(cluster="Sollwerte 1") -> (array=w322:sgl[])
        n244 = Cluster To Array(cluster="Sollwerte 3") -> (array=w324:sgl[])
        n245 = Cluster To Array(cluster="Sollwerte 2") -> (array=w323:sgl[])
        n246 = Cluster To Array(cluster="Sollwerte 4") -> (array=w303:sgl[])
        n247 = Cluster To Array(cluster="Komponenten 1") -> (array=w329:u16[])
        n248 = Cluster To Array(cluster="Komponenten 3") -> (array=w326:u16[])
        n249 = Cluster To Array(cluster="Komponenten 4") -> (array=w305:u16[])
        n250 = Cluster To Array(cluster="Komponenten 2") -> (array=w327:u16[])
        n251 = Build Path(base path="Pfad:", name or relative path=w309) -> (appended path=w308:path)
        n252 = Build Array(w318, w317, w319, w301) -> (w314:sgl[][])
        n253 = Build Array(w322, w323, w324, w303) -> (w320:sgl[][])
        n254 = Build Array(w329, w327, w326, w305) -> (w325:u16[][])
        n255 = Build Array("Analysator 1", "Analysator 2", "Analysator 3", u16 2) -> (w297:T5[])
        n256 = call "FGV CG-Check.vi"("Komponenten"=w325, "Sollwerte"=w320, "Gaskonfig"=w284, "max Abweichung"=w314, "Cluster"="Cluster", "Pfad:"=w308, "Analysator"=w297, "Aktion"=Aktion_CG-Check."schreiben") -> ("Komponenten"=w281:u16[][])  [unwired: 4 in, 7 out]
        n257 = flat-sequence {
          tunnel: w281 -> [_]
          frame #0 {
            n258 = call "FGV CG-Check.vi"("Aktion"=Aktion_CG-Check."speichern") -> ()  [unwired: 11 in, 8 out]
          }
        }
      }
      event "Abbrechen": Value Change {
        n259 = event-data() -> ()  [unwired: 1 in, 6 out]
      }
    }
  }
  n260 = flat-sequence {
    tunnel: w5 -> [_]
    frame #0 {
      n261 = vi-ref "VI CG-Check Konfig.vi"() -> (w334:refnum<vi>)
      n262 = call "VI Shut Down.vi"("VI Referenz"=w334) -> ()  [unwired: 11 in]
    }
  }
